vi "Trigger the captured image.vi"() -> ()   [LabVIEW 2009]
uses:
  D/Program Files (x86)/National Instruments/LabVIEW 2015/user.lib/LabViewDVPCamera/LabViewDVPCamera.lvlib
panel:
  out "Image":T1(plugin-control)
  in  "Trigger":bool
  in  "CloseFlg":i32
  out "handle":u32
  in  "CameraList":u16(ring) items=["USB2_1.2M_MONO(32)@UE121303030", "USB3_CMOS_16M(2)@UB16A000000"]
  in  "Set":bool
  in  "Close":bool
  in  "Open":bool
  in  "ScanCamera":bool
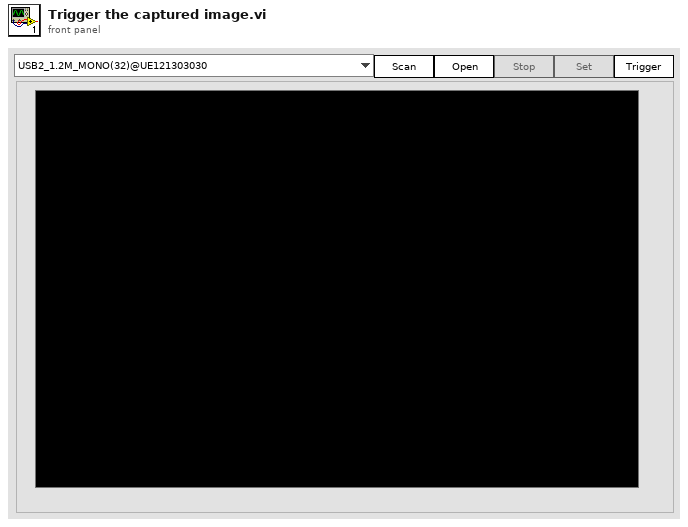
[diagram p1: front panel]
types:
  T1 = typedef "IMAQ Image.ctl" = refnum<image>
  T2 = enum8{"Enabled", "Disabled", "Disabled and Grayed Out"}
  T3 = typedef "LVStringsAndValuesArrayTypeDef_U16.ctl" = cluster{"String":string, "Value":u16}[]
  T4 = typedef "Image Type" = u32
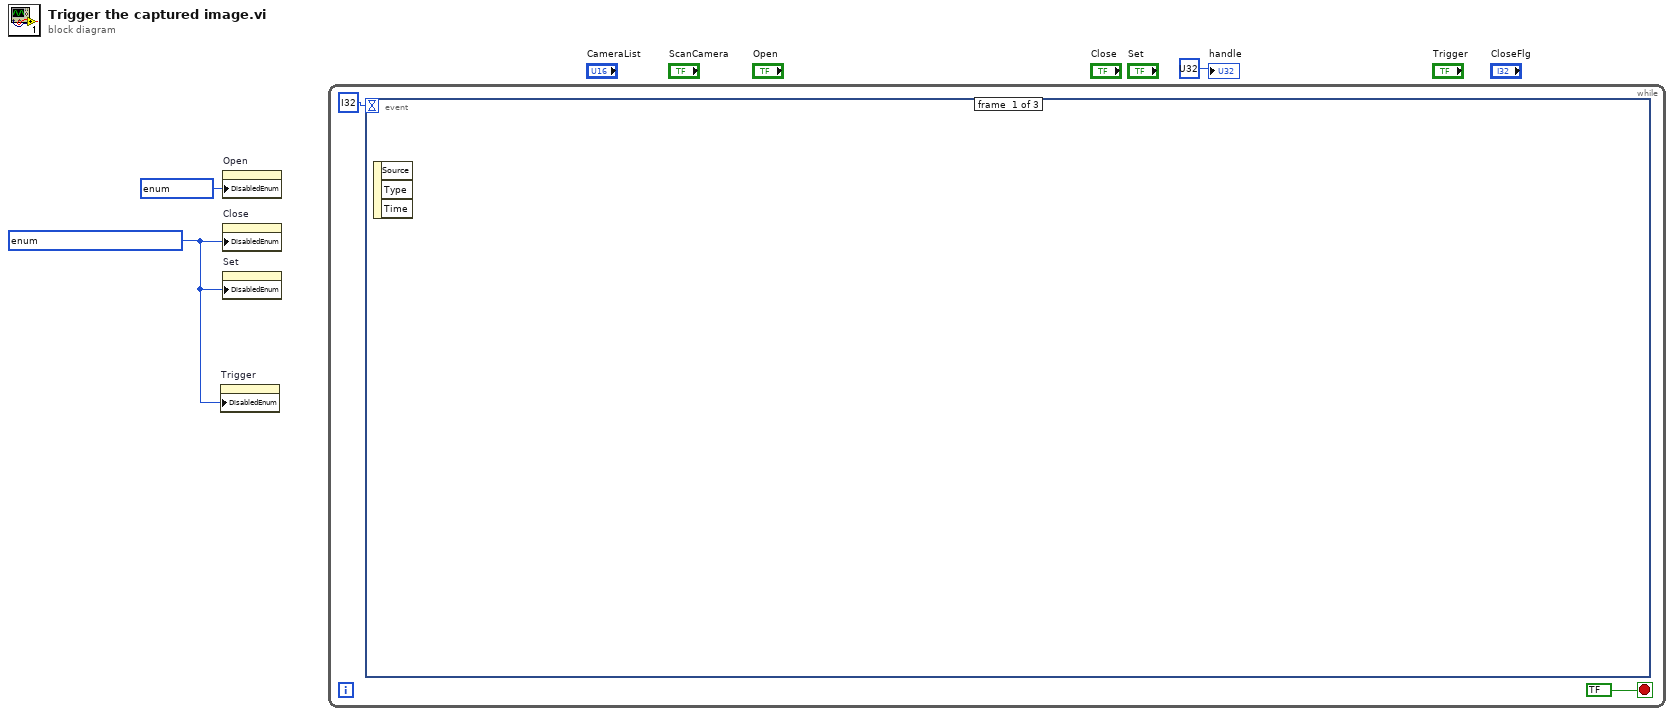
[diagram p0: block diagram]
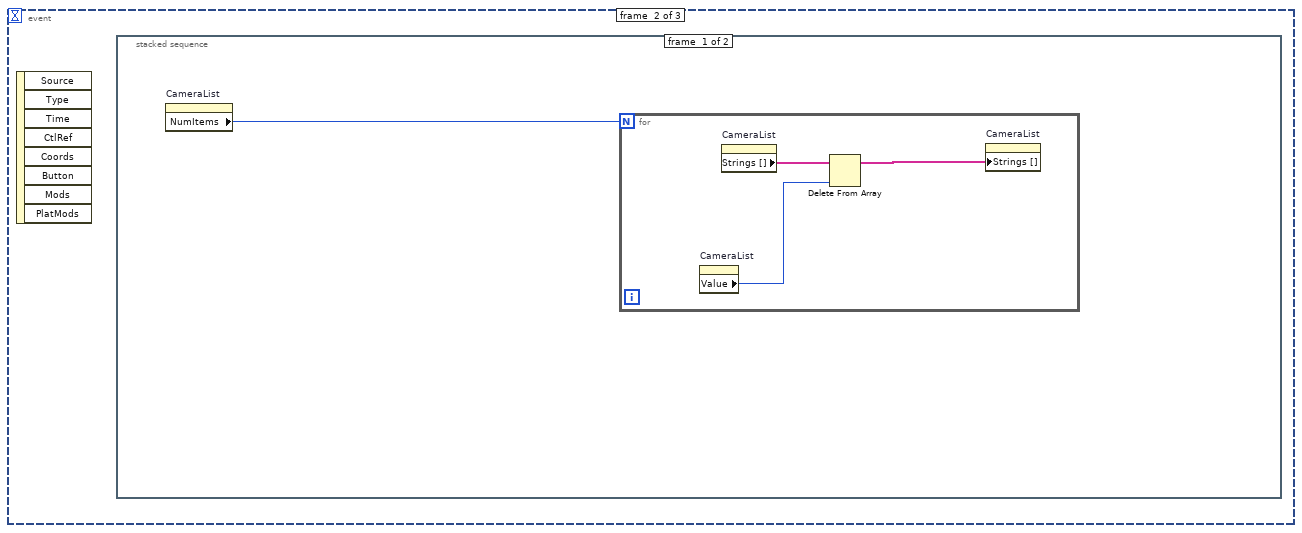
[diagram p2: hidden frame]
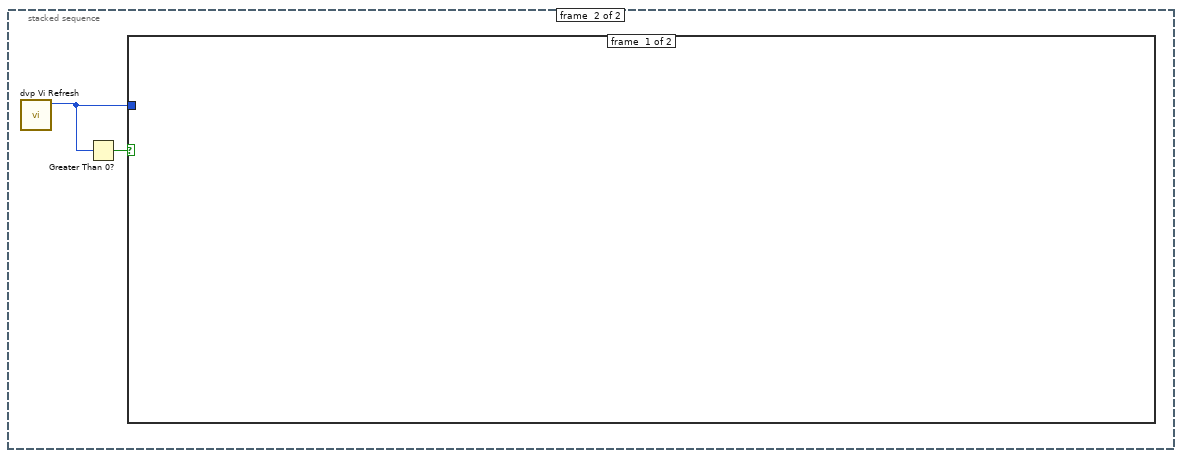
[diagram p3: hidden frame]
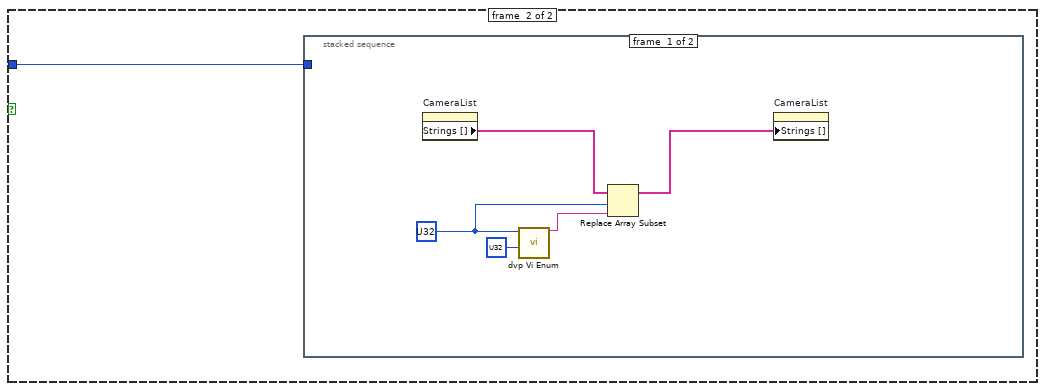
[diagram p4: hidden frame]
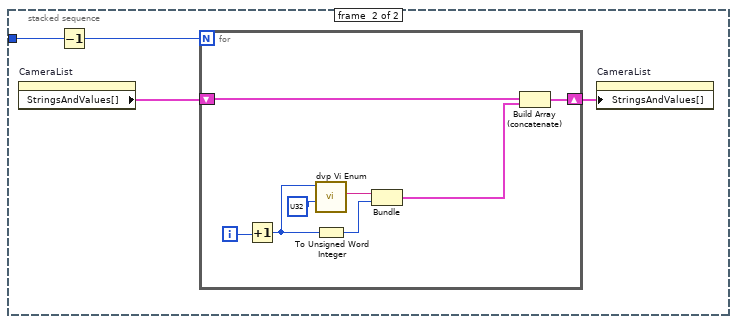
[diagram p5: hidden frame]
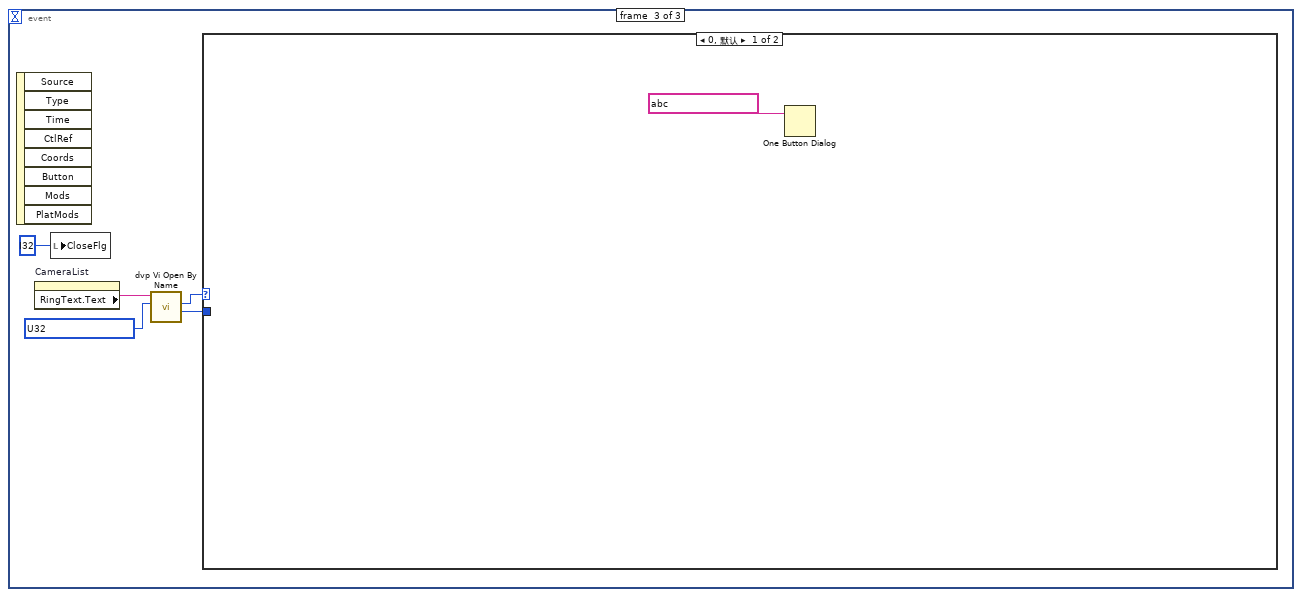
[diagram p6: hidden frame]
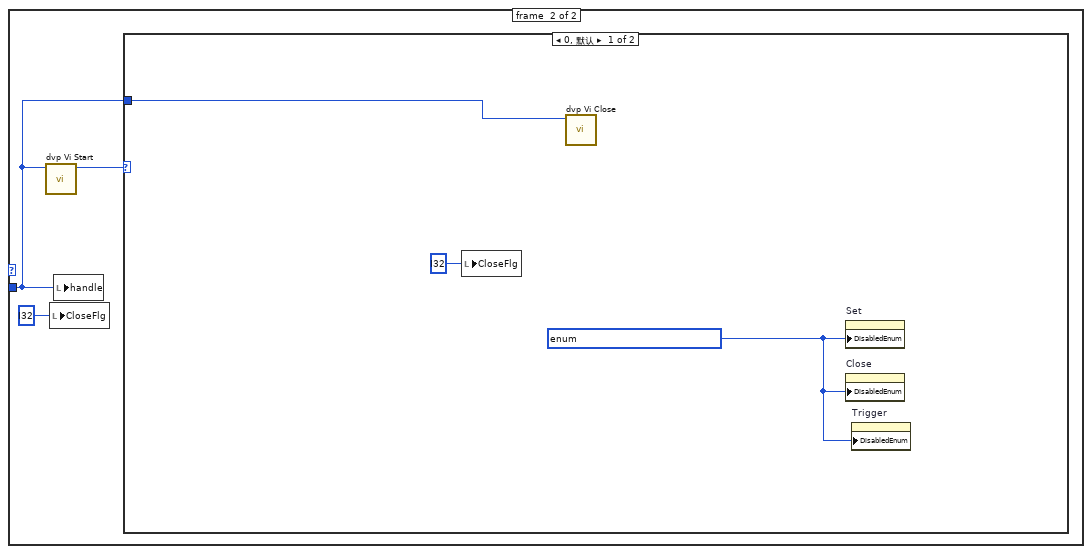
[diagram p7: hidden frame]
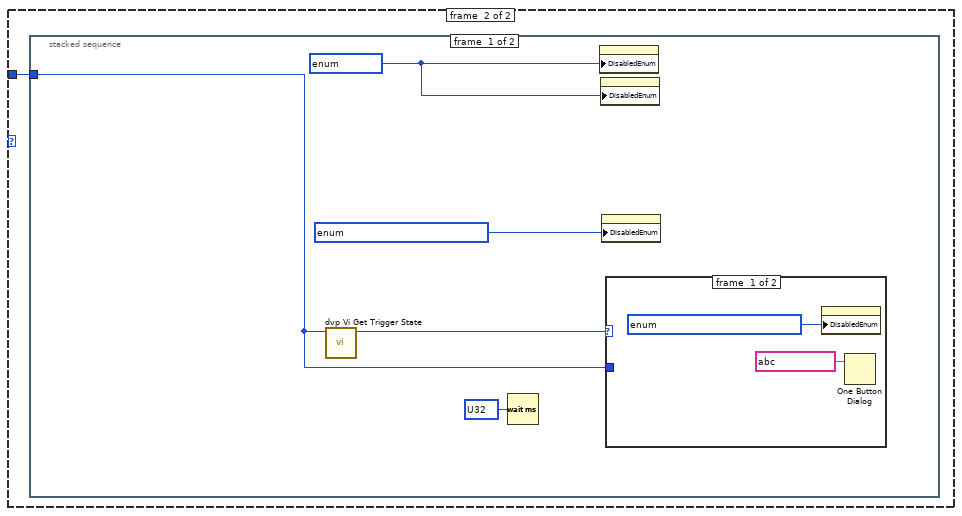
[diagram p8: hidden frame]
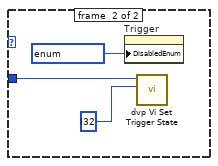
[diagram p9: hidden frame]
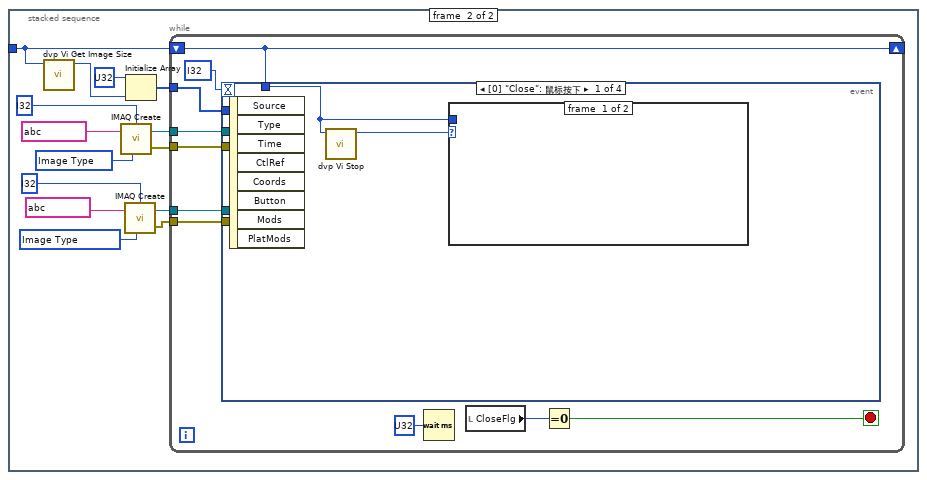
[diagram p10: hidden frame]
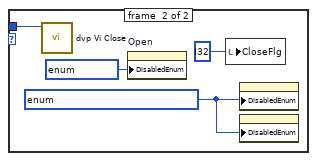
[diagram p11: hidden frame]
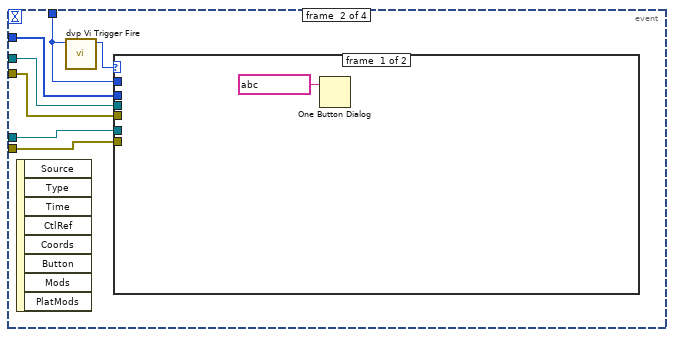
[diagram p12: hidden frame]
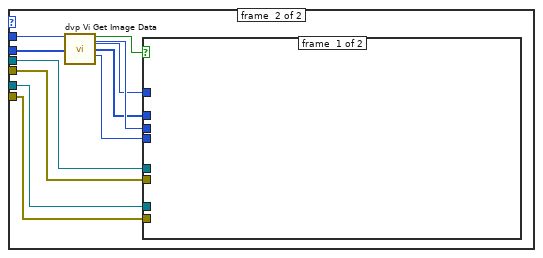
[diagram p13: hidden frame]
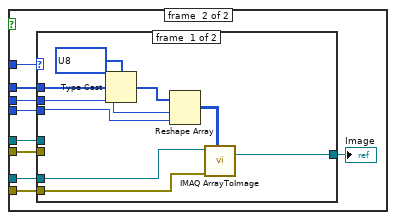
[diagram p14: hidden frame]
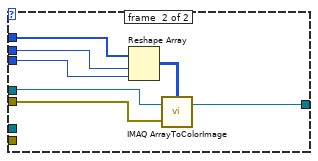
[diagram p15: hidden frame]
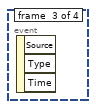
[diagram p16: hidden frame]
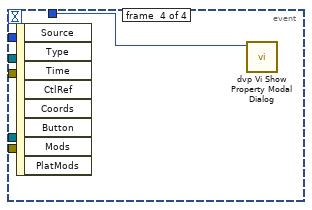
[diagram p17: hidden frame]
diagram:
  w1 = T2 ? ("禁用")
  n1 = property on="Trigger" class="Bool"("DisabledEnum"=w1) -> ()  [unwired: 2 in, 2 out]
  n2 = property on="Open" class="Bool"("DisabledEnum"=T2 ? ("禁用")) -> ()  [unwired: 2 in, 2 out]
  n3 = property on="Close" class="Bool"("DisabledEnum"=w1) -> ()  [unwired: 2 in, 2 out]
  n4 = property on="Set" class="Bool"("DisabledEnum"=w1) -> ()  [unwired: 2 in, 2 out]
  n5 = while {
    stop <- bool ? stop-if-true
    n6 = event shown="[1] \"ScanCamera\": 鼠标按下" {
      selector: _ -> [_ _ _]
      dyn-events: _ -> [_ _ _]
      timeout: i32 ? -> [_ _ _]
      event #0 {
        n7 = event-data() -> ()  [unwired: 1 in, 3 out]
      }
      event #1 {
        n8 = event-data() -> ()  [unwired: 1 in, 8 out]
        n9 = stacked-sequence "清除下拉列表的数据" {
          frame #0 {
            n10 = property on="CameraList" class="Ring (严格)"() -> ("NumItems"=w6:u32)  [unwired: 2 in, 2 out]
            n11 = for {
              N: w6 -> [_]
              n12 = property on="CameraList" class="Ring (严格)"() -> ("Value"=w8:u16)  [unwired: 2 in, 2 out]
              n13 = property on="CameraList" class="Ring (严格)"() -> ("Strings []"=w7:string[])  [unwired: 2 in, 2 out]
              n14 = Delete From Array ("删除数组元素")(array=w7, index=w8) -> (array with subset deleted=w9:string[])  [unwired: 1 in, 1 out]
              n15 = property on="CameraList" class="Ring (严格)"("Strings []"=w9) -> ()  [unwired: 2 in, 2 out]
            }
          }
          frame #1 {
            n16 = call "dvp Vi Refresh.vi"() -> ("pCount out"=w11:u32)  [unwired: 10 in, 1 out]
            n17 = Greater Than 0?(x=w11) -> (x > 0?=w10:bool)
            n18 = case shown="真" w10 {
              tunnel: w11 -> [_ w12]
              frame #0 {
              }
              frame #1 {
                n19 = stacked-sequence {
                  tunnel: w12 -> [_ w19]
                  frame #0 {
                    w13 = u32 ? ("index")
                    n20 = property on="CameraList" class="Ring (严格)"() -> ("Strings []"=w16:string[])  [unwired: 2 in, 2 out]
                    n21 = call "dvp Vi Enum.vi"("unSize"=u32 ?, "index"=w13) -> ("friendlyName out"=w15:string)  [unwired: 8 in, 1 out]
                    n22 = Replace Array Subset ("替换数组子集")(array=w16, new element=w15, index=w13) -> (w17:string[])
                    n23 = property on="CameraList" class="Ring (严格)"("Strings []"=w17) -> ()  [unwired: 2 in, 2 out]
                  }
                  frame #1 {
                    n24 = property on="CameraList" class="Ring (严格)"() -> ("StringsAndValues[]"=w21:T3)  [unwired: 2 in, 2 out]
                    n25 = Decrement(x=w19) -> (x-1=w18:u32)
                    n26 = for {
                      N: w18 -> [_]
                      shift-right: [w28] -> w20
                      shift-left: w21 -> [w26]
                      i -> [w23]
                      n27 = Increment(x=w23) -> (x+1=w22:i32)
                      n28 = call "dvp Vi Enum.vi"("unSize"=u32 ?, "index"=w22) -> ("friendlyName out"=w29:string)  [unwired: 8 in, 1 out]
                      n29 = To Unsigned Word Integer(number=w22) -> (unsigned 16bit integer=w25:u16)
                      n30 = Bundle("friendlyName out"=w29, w25) -> (w27:cluster{"friendlyName out":string, u16})  [unwired: 1 in]
                      n31 = Build Array (concatenate)(w26, w27) -> (w28:T3)
                    }
                    n32 = property on="CameraList" class="Ring (严格)"("StringsAndValues[]"=w20) -> ()  [unwired: 2 in, 2 out]
                  }
                }
              }
            }
          }
        }
      }
      event #2 {
        w32 = u32 ? items=["OPEN_OFFLINE", "OPEN_NORMAL"] ("type")
        n33 = event-data() -> ()  [unwired: 1 in, 8 out]
        n34 = property on="CameraList" class="Ring (严格)"() -> ("RingText.Text"=w31:string)  [unwired: 2 in, 2 out]
        n35 = local write "CloseFlg"(i32 ? ("CloseFlg")) -> ()
        n36 = call "dvp Vi Open By Name.vi"("type"=w32, "friendlyName"=w31) -> ("pHandle out"=w34:u32, "function return"=w33:u32)  [unwired: 7 in, 1 out]
        n37 = case shown="0, 默认" w33 {
          tunnel: w34 -> [_ w38]
          frame #0 {
            n38 = One Button Dialog(message=string ? ("消息")) -> ()  [unwired: 1 in, 1 out]
          }
          frame #1 {
            n39 = call "dvp Vi Start.vi"("handle"=w38) -> ("function return"=w36:u32)  [unwired: 10 in]
            n40 = local write "CloseFlg"(i32 ? ("CloseFlg")) -> ()
            n41 = local write "handle"(w38) -> ()
            n42 = case shown="0, 默认" w36 {
              tunnel: w38 -> [w41 w42]
              frame #0 {
                w39 = T2 ? ("禁用")
                n43 = local write "CloseFlg"(i32 ? ("CloseFlg")) -> ()
                n44 = call "dvp Vi Close.vi"("handle"=w41) -> ()  [unwired: 10 in, 1 out]
                n45 = property on="Set" class="Bool"("DisabledEnum"=w39) -> ()  [unwired: 2 in, 2 out]
                n46 = property on="Close" class="Bool"("DisabledEnum"=w39) -> ()  [unwired: 2 in, 2 out]
                n47 = property on="Trigger" class="Bool"("DisabledEnum"=w39) -> ()  [unwired: 2 in, 2 out]
              }
              frame #1 {
                n48 = stacked-sequence {
                  tunnel: w42 -> [w44 w54]
                  frame #0 {
                    w46 = T2 ? ("禁用")
                    n49 = call "dvp Vi Get Trigger State.vi"("handle"=w44) -> ("function return"=w45:u32)  [unwired: 9 in, 1 out]
                    n50 = Wait (ms)(milliseconds to wait=u32 ? ("等待时间（毫秒）")) -> ()  [unwired: 1 out]
                    n51 = property on="Set" class="Bool"("DisabledEnum"=w46) -> ()  [unwired: 2 in, 2 out]
                    n52 = property on="Close" class="Bool"("DisabledEnum"=w46) -> ()  [unwired: 2 in, 2 out]
                    n53 = property on="Open" class="Bool"("DisabledEnum"=T2 ? ("禁用")) -> ()  [unwired: 2 in, 2 out]
                    n54 = case shown="1" w45 {
                      tunnel: w44 -> [_ w51]
                      frame #0 {
                        n55 = property on="Trigger" class="Bool"("DisabledEnum"=T2 ? ("禁用")) -> ()  [unwired: 2 in, 2 out]
                        n56 = One Button Dialog(message=string ? ("消息")) -> ()  [unwired: 1 in, 1 out]
                      }
                      frame #1 {
                        n57 = property on="Trigger" class="Bool"("DisabledEnum"=T2 ? ("禁用")) -> ()  [unwired: 2 in, 2 out]
                        n58 = call "dvp Vi Set Trigger State.vi"("TriggerState"=i32 ?, "handle"=w51) -> ()  [unwired: 9 in, 1 out]
                      }
                    }
                  }
                  frame #1 {
                    w60 = T4 ? items=["Grayscale (U8)", "Grayscale (I16)", "Grayscale (SGL)", "Complex (CSG)", "RGB (U32)", "HSL (U32)", "RGB (U64)", "Grayscale (U16)"] ("Image Type")
                    w64 = T4 ? items=["Grayscale (U8)", "Grayscale (I16)", "Grayscale (SGL)", "Complex (CSG)", "RGB (U32)", "HSL (U32)", "RGB (U64)", "Grayscale (U16)"] ("Image Type")
                    n59 = call "dvp Vi Get Image Size.vi"("handle"=w54) -> ("function return"=w65:u32)  [unwired: 10 in]
                    n60 = call "IMAQ Create"("Border Size"=i32 ?, "Image Name"=string ?, "Image Type"=w64) -> ("New Image"=w56:T1, "error out"=w55:errorcluster)  [unwired: 2 in]
                    n61 = call "IMAQ Create"("Border Size"=i32 ?, "Image Name"=string ?, "Image Type"=w60) -> ("New Image"=w53:T1, "error out"=w57:errorcluster)  [unwired: 2 in]
                    n62 = Initialize Array(u32 ? ("元素"), w65) -> (w58:u32[])
                    n63 = while {
                      shift-right: [w72] -> _
                      shift-left: w54 -> [w72]
                      tunnel: w58 -> [w71]
                      tunnel: w57 -> [w67]
                      tunnel: w56 -> [w70]
                      tunnel: w55 -> [w69]
                      tunnel: w53 -> [w68]
                      stop <- w75 stop-if-true
                      n64 = event shown="[0] \"Close\": 鼠标按下" {
                        selector: _ -> [_ _ _ _]
                        dyn-events: _ -> [_ _ _ _]
                        timeout: i32 ? -> [_ _ _ _]
                        tunnel: w72 -> [w77 w88 _ w127]
                        tunnel: w71 -> [_ w87 _ _]
                        tunnel: w70 -> [_ w84 _ _]
                        tunnel: w69 -> [_ w83 _ _]
                        tunnel: w68 -> [_ w86 _ _]
                        tunnel: w67 -> [_ w85 _ _]
                        event #0 {
                          n65 = event-data() -> ()  [unwired: 1 in, 8 out]
                          n66 = call "dvp Vi Stop.vi"("handle"=w77) -> ("function return"=w78:u32)  [unwired: 10 in]
                          n67 = case shown="1" w78 {
                            tunnel: w77 -> [_ w80]
                            frame #0 {
                            }
                            frame #1 {
                              w79 = T2 ? ("禁用")
                              n68 = call "dvp Vi Close.vi"("handle"=w80) -> ()  [unwired: 10 in, 1 out]
                              n69 = property on="Open" class="Bool"("DisabledEnum"=T2 ? ("禁用")) -> ()  [unwired: 2 in, 2 out]
                              n70 = local write "CloseFlg"(i32 ? ("CloseFlg")) -> ()
                              n71 = property on="Close" class="Bool"("DisabledEnum"=w79) -> ()  [unwired: 2 in, 2 out]
                              n72 = property on="Set" class="Bool"("DisabledEnum"=w79) -> ()  [unwired: 2 in, 2 out]
                            }
                          }
                        }
                        event #1 {
                          n73 = event-data() -> ()  [unwired: 1 in, 8 out]
                          n74 = call "dvp Vi Trigger Fire.vi"("handle"=w88) -> ("function return"=w89:u32)  [unwired: 10 in]
                          n75 = case shown="1" w89 {
                            tunnel: w88 -> [_ w96]
                            tunnel: w87 -> [_ w91]
                            tunnel: w86 -> [_ w93]
                            tunnel: w85 -> [_ w92]
                            tunnel: w84 -> [_ w95]
                            tunnel: w83 -> [_ w94]
                            frame #0 {
                              n76 = One Button Dialog(message=string ? ("消息")) -> ()  [unwired: 1 in, 1 out]
                            }
                            frame #1 {
                              n77 = call "dvp Vi Get Image Data.vi"("handle"=w96, "pbuffer"=w91) -> ("piHeight out"=w100:i32, "function return"=w97:bool, "pformat out"=w98:i32, "pbuffer out"=w99:u32[], "piWidth out"=w101:i32)  [unwired: 9 in]
                              n78 = case shown="真" w97 {
                                tunnel: w101 -> [_ w110]
                                tunnel: w100 -> [_ w109]
                                tunnel: w99 -> [_ w108]
                                tunnel: w98 -> [_ w107]
                                tunnel: w95 -> [_ w103]
                                tunnel: w93 -> [_ w106]
                                tunnel: w92 -> [_ w105]
                                tunnel: w94 -> [_ w104]
                                frame #0 {
                                }
                                frame #1 {
                                n79 = case shown="1" w107 {
                                tunnel: w109 -> [w119 w125]
                                tunnel: w110 -> [w118 w126]
                                tunnel: [w117 w123] -> w102
                                tunnel: w108 -> [w114 w122]
                                tunnel: w106 -> [w111 _]
                                tunnel: w105 -> [w112 _]
                                tunnel: w104 -> [_ w120]
                                tunnel: w103 -> [_ w121]
                                frame #0 {
                                n80 = Type Cast(type=u8[] ?, x=w114) -> (*(type *) &x=w113:u8[])
                                n81 = Reshape Array ("重排数组维数")(w113, w119, w118) -> (w116:u8[][])
                                n82 = call "IMAQ ArrayToImage"("error in (no error)"=w112, "Image Pixels (U8)"=w116, "Image"=w111) -> ("Image Out"=w117:T1)  [unwired: 7 in, 1 out]
                                }
                                frame #1 {
                                n83 = Reshape Array ("重排数组维数")(w122, w125, w126) -> (w124:u32[][])
                                n84 = call "IMAQ ArrayToColorImage"("Image Pixels (U32)"=w124, "Image"=w121, "error in (no error)"=w120) -> ("Image Out"=w123:T1)  [unwired: 2 in, 1 out]
                                }
                                }
                                "Image" <- w102
                                }
                              }
                            }
                          }
                        }
                        event #2 {
                          n85 = event-data() -> ()  [unwired: 1 in, 3 out]
                        }
                        event #3 {
                          n86 = event-data() -> ()  [unwired: 1 in, 8 out]
                          n87 = call "dvp Vi Show Property Modal Dialog.vi"("handle"=w127) -> ()  [unwired: 10 in, 1 out]
                        }
                      }
                      n88 = Wait (ms)(milliseconds to wait=u32 ? ("等待时间（毫秒）")) -> ()  [unwired: 1 out]
                      n89 = local read "CloseFlg"() -> (w74:i32)
                      n90 = Equal To 0?(x=w74) -> (x = 0?=w75:bool)
                    }
                  }
                }
              }
            }
          }
        }
      }
    }
  }
  "handle" <- u32 ? ("handle")
